vi "TestRayTriInter.vi"() -> ()   [LabVIEW 2014]
uses:
  TypeDefs/TriangleFace.ctl
  TypeDefs/Point3D.ctl
panel:
  out "P0":T1
  out "Intersects":bool
  out "r":dbl
  in  "Ray":T2
  in  "TriangleFace":T3
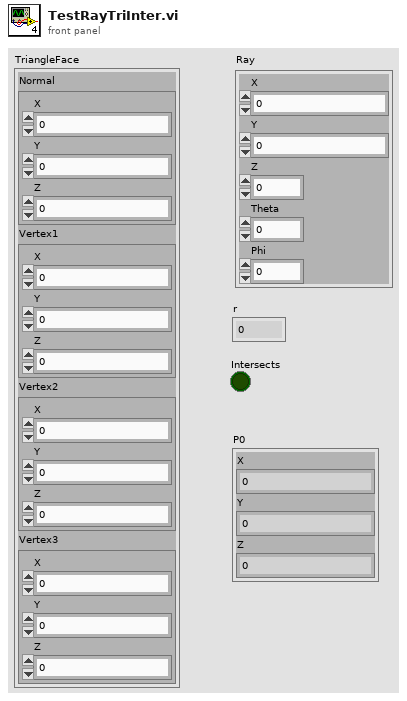
[diagram p1: front panel]
types:
  T1 = typedef "Point3D.ctl" = cluster{"X":sgl, "Y":sgl, "Z":sgl}
  T2 = cluster{"X":dbl, "Y":dbl, "Z":dbl, "Theta":dbl, "Phi":dbl}
  T3 = typedef "TriangleFace.ctl" = cluster{"Normal":T1, "Vertex1":T1, "Vertex2":T1, "Vertex3":T1}
  T4 = cluster{"P0":cluster{"X":dbl, "Y":dbl, "Z":dbl}, "P0":cluster{"X":dbl, "Y":dbl, "Z":dbl}}
  T5 = cluster{"P0":cluster{"X":dbl, "Y":dbl, "Z":dbl}, "P0":cluster{"X":dbl, "Y":dbl, "Z":dbl}}[]
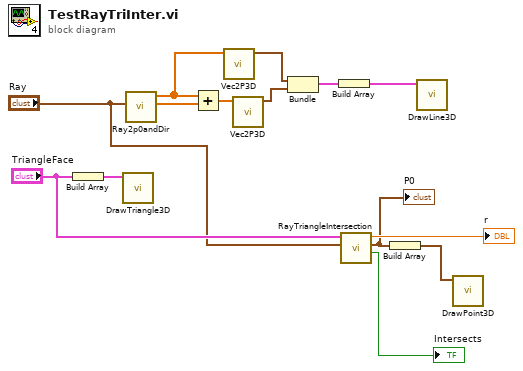
[diagram p0: block diagram]
diagram:
  n1 = Build Array("TriangleFace") -> (w7:T3[])
  n2 = call "DrawTriangle3D.vi"("Triangles"=w7) -> ()  [unwired: 11 in]
  n3 = call "Ray2p0andDir.vi"("Ray"="Ray") -> ("Dir"=w14:dbl[], "P0"=w11:dbl[])  [unwired: 9 in]
  n4 = Add(x=w11, y=w14) -> (x+y=w9:dbl[])
  n5 = call "Vec2P3D.vi"("Vec"=w11) -> ("P0"=w10:cluster{"X":dbl, "Y":dbl, "Z":dbl})  [unwired: 10 in]
  n6 = call "Vec2P3D.vi"("Vec"=w9) -> ("P0"=w8:cluster{"X":dbl, "Y":dbl, "Z":dbl})  [unwired: 10 in]
  n7 = Bundle("P0"=w10, "P0"=w8) -> (w13:T4)  [unwired: 1 in]
  n8 = Build Array(w13) -> (w12:T5)
  n9 = call "RayTriangleIntersection.vi"("Ray"="Ray", "TriangleFace"="TriangleFace") -> ("Intersects"=→"Intersects":bool, "P0"=w3:cluster{"X":dbl, "Y":dbl, "Z":dbl}, "r"=→"r":dbl)  [unwired: 7 in]
  "P0" <- w3
  n10 = Build Array(w3) -> (w2:cluster{"X":dbl, "Y":dbl, "Z":dbl}[])
  n11 = call "DrawLine3D.vi"("Lines"=w12) -> ()  [unwired: 11 in]
  n12 = call "DrawPoint3D.vi"("Points"=w2) -> ()  [unwired: 11 in]
